vi "Post_Build_Windows.vi"(8 "error in (no error)":errorcluster, 11 "Destination Path":path) -> (0 "error out":errorcluster, 3 "Zip File":path)   [LabVIEW 2017]
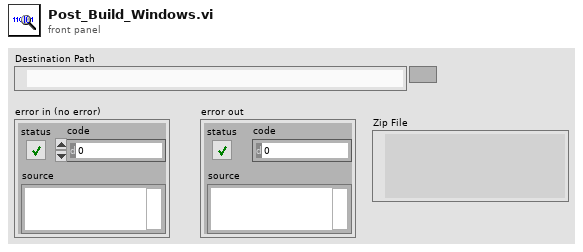
[diagram p1: front panel]
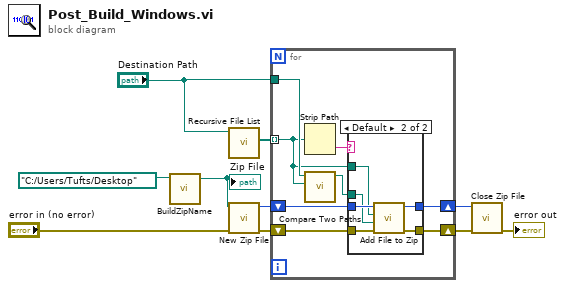
[diagram p0: block diagram]
diagram:
  n1 = call "BuildZipName.vi"("Folder"=path "C:/Users/Tufts/Desktop" ("target")) -> ("Zip File"=w1:path)  [unwired: 10 in]
  "Zip File" <- w1
  n2 = call <vilib>:"Recursive File List.vi"("Folder Path"="Destination Path") -> ("All Files in Dir"=w6:path[])  [unwired: 6 in, 4 out]
  n3 = call <vilib>:"New Zip File.vi"("error in (no error)"="error in (no error)", "target"=w1) -> ("error out"=w8:errorcluster, "zip file out"=w4:i64)  [unwired: 3 in, 1 out]
  n4 = for {
    tunnel: w6 -> [w13] mode=indexing
    shift-right: [w17] -> w5
    shift-left: w4 -> [w18]
    tunnel: "Destination Path" -> [w14]
    shift-right: [w11] -> w9
    shift-left: w8 -> [w12]
    n5 = Strip Path(path=w13) -> (name=w16:string)  [unwired: 1 out]
    n6 = call <vilib>:"Compare Two Paths.vi"("Path 2"=w13, "Path 1"=w14) -> ("Relative Path from 1 to 2"=w15:path)  [unwired: 6 in, 3 out]
    n7 = case shown="Default" w16 {
      tunnel: w13 -> [_ w24]
      tunnel: w18 -> [w20 w26]
      tunnel: [w20 w25] -> w17
      tunnel: w15 -> [_ w23]
      tunnel: w12 -> [w19 w22]
      tunnel: [w19 w21] -> w11
      frame ".DS_Store" {
      }
      frame Default {
        n8 = call <vilib>:"Add File to Zip.vi"("error in (no error)"=w22, "destination path in zip"=w23, "source file path"=w24, "zip file in"=w26) -> ("error out"=w21:errorcluster, "zip file out"=w25:i64)  [unwired: 6 in]
      }
    }
  }
  n9 = call <vilib>:"Close Zip File.vi"("error in (no error)"=w9, "zip file in"=w5) -> ("error out"=→"error out":errorcluster)  [unwired: 5 in]
